vi "Stop Core.vi"(10 "final error code":i32, 11 "Application in":refnum<class "Application.lvclass">) -> (3 "Application out":refnum<class "Application.lvclass">)   [LabVIEW 2023, in "Application.lvlib" / "Application.lvclass"]
doc: "(<B>Filename</B>: Actor Framework.lvlib:Actor.lvclass:Stop Core.vi)\n\nDefines what the actor does before it stops. Use the <B>final error code</B> input to determine whether the actor shut down in response to an error.\n\nBy default, this method passes the Stop message along to all auto-stop nested actors. A descendant class may override this method to define additional behavior, such as shutting down any processes the actor initiated in its override of the Actor Core method."
uses:
  Application.lvclass
  Mode.ctl
  Application.lvclass/Application.ctl
  <vilib>/ActorFramework/Actor/Actor.lvclass
  Application.lvlib
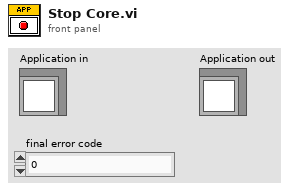
[diagram p1: front panel]
types:
  T1 = typedef "Application.lvlib/Mode.ctl" = enum16{"Idle", "Cancel", "Live", "Stream", "Autofocus", "Z-Stack"}
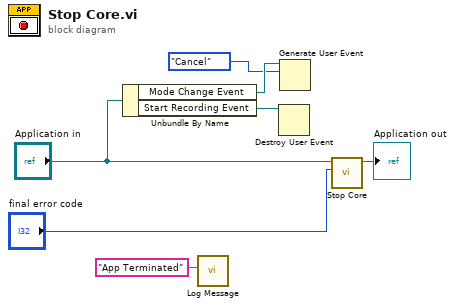
[diagram p0: block diagram]
diagram:
  n1 = Unbundle By Name("Application in") -> ("Mode Change Event"=w3:refnum<user-event>, "Start Recording Event"=w4:refnum<user-event>)
  n2 = call "Log Message.vi"("input"="App Terminated") -> ()  [unwired: 9 in, 2 out]
  n3 = Destroy User Event(user event=w4) -> ()  [unwired: 1 in, 1 out]
  n4 = Generate User Event(user event=w3, event data cluster=Mode."Cancel" ("Mode")) -> ()  [unwired: 2 in, 2 out]
  n5 = call-parent "Stop Core.vi"("final error code"="final error code", "Actor in"="Application in") -> ("Actor out"=→"Application out":refnum<class "Application.lvclass">)  [unwired: 9 in]
